vi "get_average_photodiode_voltage.vi"(7 "number of reads":i32=1, 8 "error in (no error)":errorcluster) -> (0 "error out":errorcluster, 3 "voltage":dbl format="%_4g")   [LabVIEW 2015]
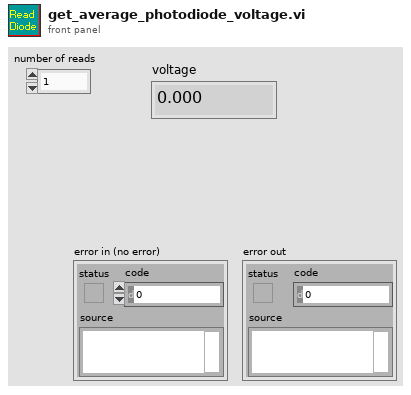
[diagram p1: front panel]
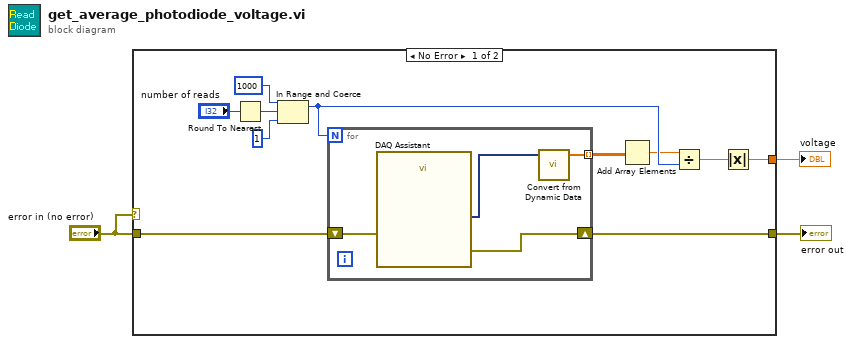
[diagram p0: block diagram]
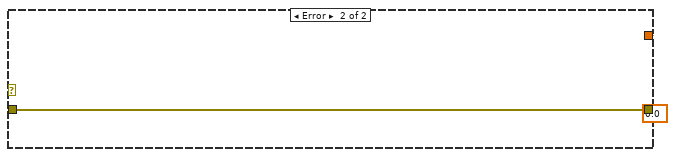
[diagram p2: hidden frame]
diagram:
  n1 = case shown="No Error" "error in (no error)" {
    tunnel: [w14 0.0] -> w2
    tunnel: "error in (no error)" -> [w6 w20]
    tunnel: [w5 w20] -> w3
    frame No Error {
      n2 = Round To Nearest(number="number of reads") -> (nearest integer value=w12:i32)
      n3 = In Range and Coerce(upper limit=1000, x=w12, lower limit=1) -> (coerced(x)=w9:i32)  [unwired: 1 out]
      n4 = for {
        N: w9 -> [_]
        shift-right: [w17] -> w5
        shift-left: w6 -> [w18]
        tunnel: [w16] -> w4 mode=indexing
        n5 = call "DAQ Assistant"("error in"=w18) -> ("data"=w15:dynamicdata, "error out"=w17:errorcluster)  [unwired: 16 in, 1 out]
        n6 = call "Convert from Dynamic Data"("Dynamic Data Type"=w15) -> ("Array"=w16:dbl[])  [unwired: 3 in]
      }
      n7 = Add Array Elements(numeric array=w4) -> (sum=w8:dbl)
      n8 = Divide(x=w8, y=w9) -> (x/y=w7:dbl)
      n9 = Absolute Value(x=w7) -> (abs(x)=w14:dbl)
    }
    frame Error {
    }
  }
  "error out" <- w3
  "voltage" <- w2
